vi "vi server test1.vi"() -> ()   [LabVIEW 2019]
panel:
  out "error out 2":errorcluster
  out "Value":variant
  in  "Control Name":string
  in  "Type":enum16{"Both", "Controls", "Indicators"}(ring)
  out "All Controls":refnum<vi>[](array[refnum])
  in  "port number or service name (3363)":u16=3375
  in  "vi path":path=path "nanocal-frontend-client-standalone-18.vi"
  in  "machine name (\"\":  open local reference)":string="TAGLIATELLE.ad.magnet.fsu.edu"
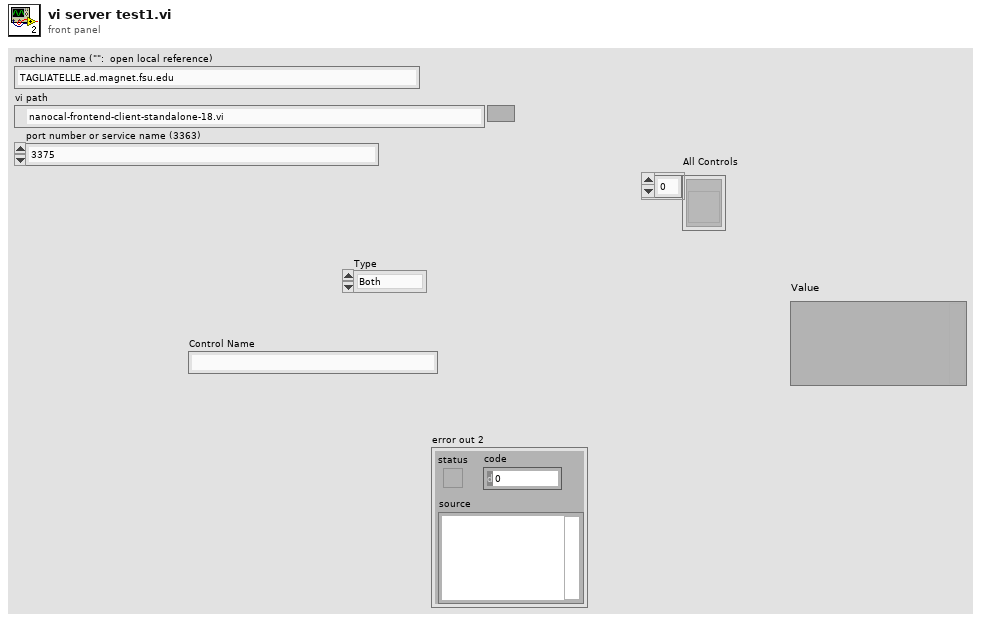
[diagram p1: front panel]
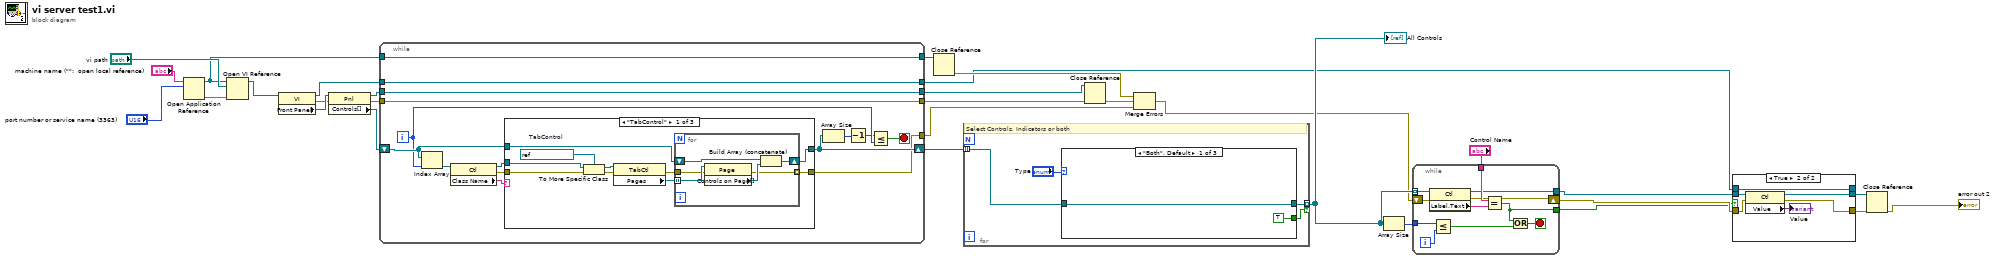
[diagram p0: block diagram]
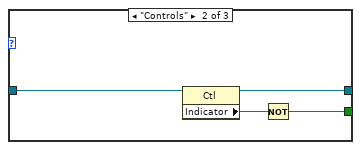
[diagram p3: hidden frame]
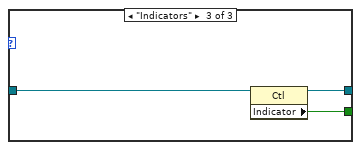
[diagram p4: hidden frame]
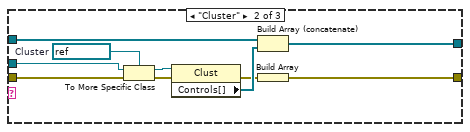
[diagram p5: hidden frame]
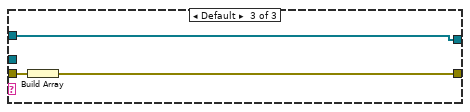
[diagram p6: hidden frame]
diagram:
  n1 = Open Application Reference(10:"port number or service name (3363)", 11:"machine name (\"\":  open local reference)") -> (0:w30:errorcluster, 3:w13:refnum<vi>)  [unwired: 2 in]
  n2 = Open VI Reference(application reference (local)=w13, vi path="vi path", error in (no error)=w30) -> (vi reference=w12:refnum<vi>)  [unwired: 3 in, 1 out]
  n3 = property class="VI"(reference=w12) -> (reference out=w17:refnum<vi>, error out=w22:errorcluster, "Front Panel"=w26:refnum<vi>)  [unwired: 1 in]
  n4 = property class="Pnl"(reference=w26, error in=w22) -> (reference out=w20:refnum<vi>, error out=w18:errorcluster, "Controls[]"=w25:refnum<vi>[])
  n5 = while {
    shift-right: [w44] -> w15
    shift-left: w25 -> [w45]
    tunnel: [w35] -> w24
    tunnel: [w34] -> w21
    tunnel: w20 -> [w34]
    tunnel: w18 -> [w33]
    tunnel: [w33] -> w19
    tunnel: w17 -> [w32]
    tunnel: [w32] -> w2
    tunnel: [w31] -> w16
    tunnel: w13 -> [w31]
    i -> [w42]
    stop <- w41 stop-if-true
    n6 = Index Array(array=w45, index=w42) -> (element=w39:refnum<vi>)
    n7 = property class="Ctl"(reference=w39) -> (reference out=w37:refnum<vi>, error out=w36:errorcluster, "Class Name"=w38:string)  [unwired: 1 in]
    n8 = case shown="\"TabControl\"" w38 {
      tunnel: w45 -> [w54 w71 w74]
      tunnel: [w53 w70 w74] -> w44
      tunnel: w37 -> [w52 w69 _]
      tunnel: w36 -> [w51 w68 w73]
      tunnel: [w46 w62 w72] -> w35
      frame "TabControl" {
        w48 = refnum<vi> refnum  # TabControl
        n9 = To More Specific Class(target class=w48, reference=w52, error in=w51) -> (specific class reference=w49:refnum<vi>, error out=w50:errorcluster)
        n10 = property class="TabCtl"(reference=w49, error in=w50) -> (error out=w47:errorcluster, "Pages"=w55:refnum<vi>[])  [unwired: 1 out]
        n11 = for {
          tunnel: w55 -> [w61] mode=indexing
          shift-right: [w60] -> w53
          shift-left: w54 -> [w59]
          tunnel: w47 -> [w57]
          tunnel: [w56] -> w46 mode=indexing
          n12 = property class="Page"(reference=w61, error in=w57) -> (error out=w56:errorcluster, "Controls on Page[]"=w58:refnum<vi>[])  [unwired: 1 out]
          n13 = Build Array (concatenate)(w59, w58) -> (w60:refnum<vi>[])
        }
      }
      frame "Cluster" {
        w65 = refnum<vi> refnum  # Cluster
        n14 = To More Specific Class(target class=w65, reference=w69, error in=w68) -> (specific class reference=w66:refnum<vi>, error out=w67:errorcluster)
        n15 = property class="Clust"(reference=w66, error in=w67) -> (error out=w63:errorcluster, "Controls[]"=w64:refnum<vi>[])  [unwired: 1 out]
        n16 = Build Array (concatenate)(w71, w64) -> (w70:refnum<vi>[])
        n17 = Build Array(w63) -> (w62:errorcluster[])
      }
      frame Default {
        n18 = Build Array(w73) -> (w72:errorcluster[])
      }
    }
    n19 = Array Size(array=w44) -> (size(s)=w43:i32)
    n20 = Decrement(x=w43) -> (x-1=w40:i32)
    n21 = Less Or Equal?(x=w40, y=w42) -> (x <= y?=w41:bool)
  }
  n22 = Close Reference(reference=w16) -> (error out=w14:errorcluster)  [unwired: 1 in]
  n23 = for {
    tunnel: w15 -> [w78] mode=indexing
    tunnel: [w77] -> w4 mode=indexing if=w76
    # "Select Controls, Indicators or both"
    n24 = case shown="\"Both\", Default" "Type" {
      tunnel: w78 -> [w80 w84 w87]
      tunnel: [w80 w83 w86] -> w77
      tunnel: [TRUE ("Indicator") w81 w85] -> w76
      frame "Both", Default {
      }
      frame "Controls" {
        n25 = property class="Ctl"(reference=w84) -> (reference out=w83:refnum<vi>, "Indicator"=w82:bool)  [unwired: 1 in, 1 out]
        n26 = Not(x=w82) -> (.not. x?=w81:bool)
      }
      frame "Indicators" {
        n27 = property class="Ctl"(reference=w87) -> (reference out=w86:refnum<vi>, "Indicator"=w85:bool)  [unwired: 1 in, 1 out]
      }
    }
  }
  "All Controls" <- w4
  n28 = Close Reference(reference=w21, error in (no error)=w19) -> (error out=w23:errorcluster)
  n29 = Merge Errors(w14, w23, w24) -> (w3:errorcluster)
  n30 = Array Size(array=w4) -> (size(s)=w10:i32)
  n31 = while {
    tunnel: w4 -> [w96] mode=indexing
    tunnel: w10 -> [w97]
    tunnel: "Control Name" -> [w94]
    tunnel: [w91] -> w7
    tunnel: [w90] -> w5
    shift-right: [w88] -> w6
    shift-left: w3 -> [w89]
    i -> [w98]
    stop <- w93 stop-if-true
    n32 = property class="Ctl"(reference=w96, error in=w89) -> (reference out=w91:refnum<vi>, error out=w88:errorcluster, "Label.Text"=w95:string)
    n33 = Less Or Equal?(x=w97, y=w98) -> (x <= y?=w92:bool)
    n34 = Equal?(x=w94, y=w95) -> (x = y?=w90:bool)
    n35 = Or(x=w90, y=w92) -> (x .or. y?=w93:bool)
  }
  n36 = case shown="True" w5 {
    tunnel: w7 -> [w100 w107]
    tunnel: [w100 w106] -> w9
    tunnel: [w101 w105] -> w8
    tunnel: w6 -> [w101 w104]
    tunnel: w2 -> [w99 w103]
    tunnel: [w99 w103] -> _
    frame False {
    }
    frame True {
      n37 = property class="Ctl"(reference=w107, error in=w104) -> (reference out=w106:refnum<vi>, error out=w105:errorcluster, "Value"=→"Value":variant)
    }
  }
  n38 = Close Reference(reference=w9, error in (no error)=w8) -> (error out=→"error out 2":errorcluster)
